vi "VXM_open_port_win7.vi"(0 "error in (no error)":errorcluster) -> (1 "VISA resource name out":refnum<visa-resource-name>, 2 "error out":errorcluster)   [LabVIEW 2017]
uses:
  <vilib>/Instr/_visa.llb/VISA Configure Serial Port (Instr).vi
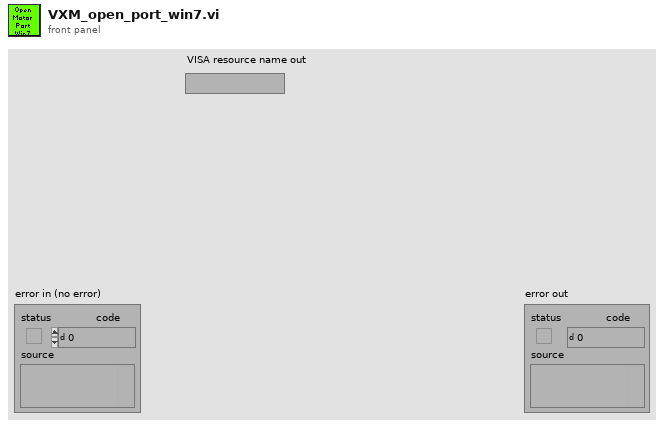
[diagram p1: front panel]
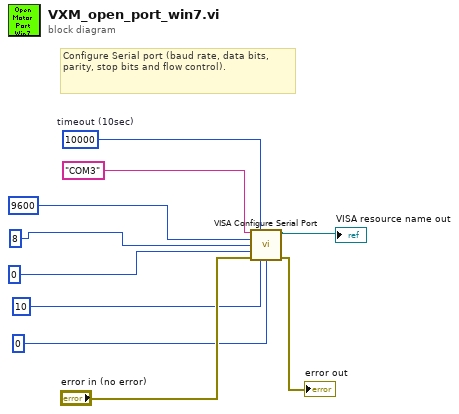
[diagram p0: block diagram]
diagram:
  w10 = u32 10000  # timeout (10sec)
  # "Configure Serial port (baud rate, data bits, parity, stop bits and flow control)."
  n1 = call-poly "VISA Configure Serial Port"("VISA resource name"="COM3", "timeout (10sec)"=w10, "baud rate (9600)"=9600, "data bits (8)"=8, "parity (0:none)"=0, "error in (no error)"="error in (no error)", "stop bits (10: 1 bit)"=10, "flow control (0:none)"=0) -> ("VISA resource name out"=→"VISA resource name out":refnum<visa-resource-name>, "error out"=→"error out":errorcluster)  [unwired: 1 in, 5 out]
